vi "From DateTime.vi"(1 "DateTime":timestamp) -> (0 "Formatted DateTime":dbl)   [LabVIEW 2013, in "OPC UA Client runtime.lvclass"]
doc: "Convert DateTime to data type which can be used by DCAF"
uses:
  OPC UA Client runtime.lvclass
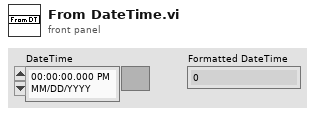
[diagram p1: front panel]
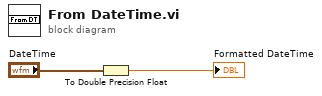
[diagram p0: block diagram]
diagram:
  n1 = To Double Precision Float(number="DateTime") -> (double precision float=→"Formatted DateTime":dbl)
